vi "Get ID Collum.vi"(8 "error in (no error)":errorcluster caption="错误输入（无错误）", 11 "ExcelSave 输入":refnum<class "ExcelSave.lvclass"> caption="DNL_LabVIEW Object in") -> (0 "error out":errorcluster caption="错误输出", 1 "ID Row":i32, 2 "ID Collum":i32, 3 "ExcelSave 输出":refnum<class "ExcelSave.lvclass"> caption="DNL_LabVIEW Object out")   [LabVIEW 2016, in "ExcelSave.lvclass"]
uses:
  ExcelSave.lvclass
  ExcelSave.lvclass/ExcelSave.ctl
  <vilib>/Utility/NIReport.llb/NI_report.lvclass
  <vilib>/addons/_office/NI_ReportGenerationToolkit.lvlib
  <vilib>/Utility/NIReport.llb/Excel/NI_Excel.lvclass
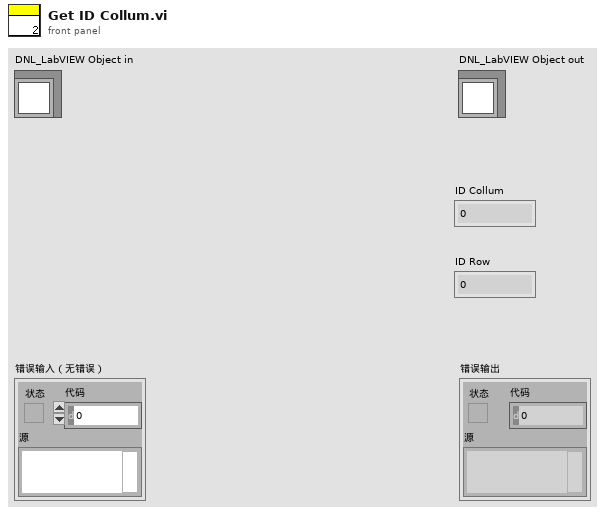
[diagram p1: front panel]
types:
  T1 = typedef "NI_ReportGenerationCore.lvlib/Report Data Members.ctl" = cluster{"font":T2, "from template?":bool}
  T2 = typedef "NI_ReportGenerationCore.lvlib/font.ctl" = cluster{"font name":string, "font size":dbl, "bold":u16, "italic":u16, "underline":u16, "strike through":u16, "font color":u32}
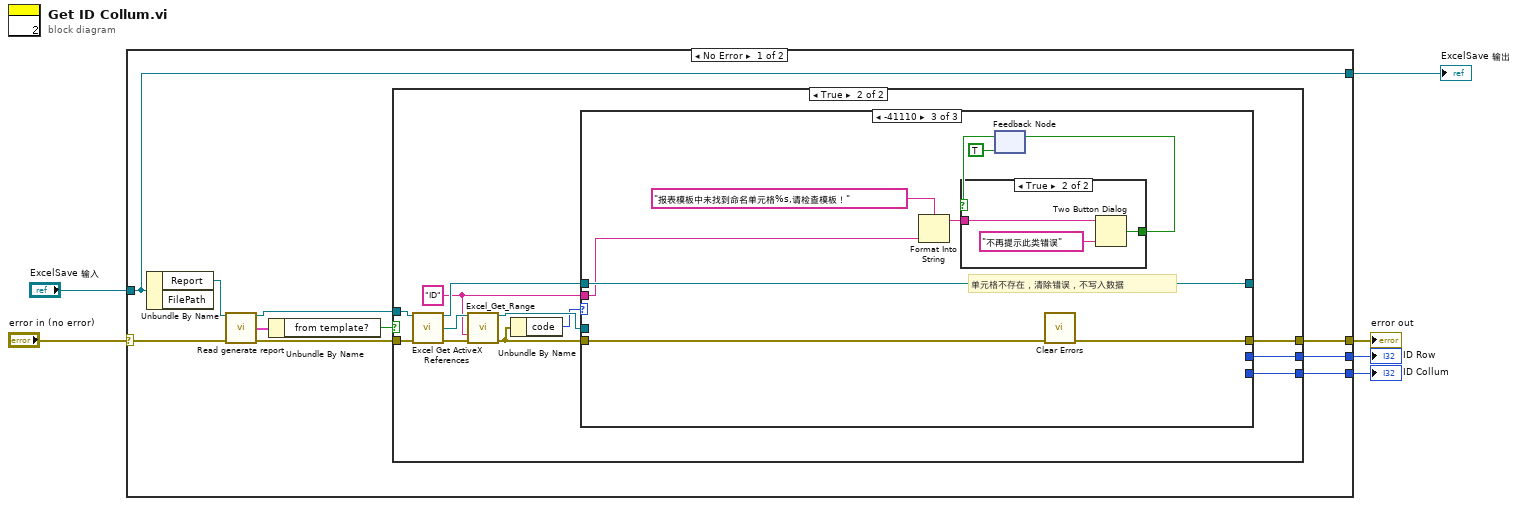
[diagram p0: block diagram]
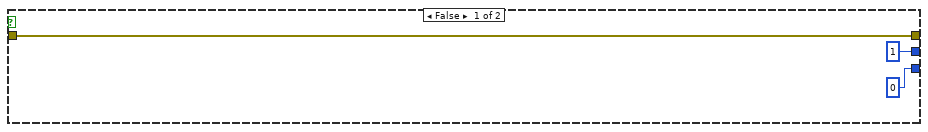
[diagram p2: hidden frame]
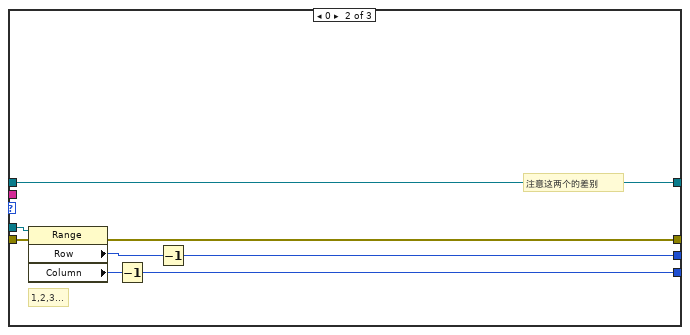
[diagram p4: hidden frame]
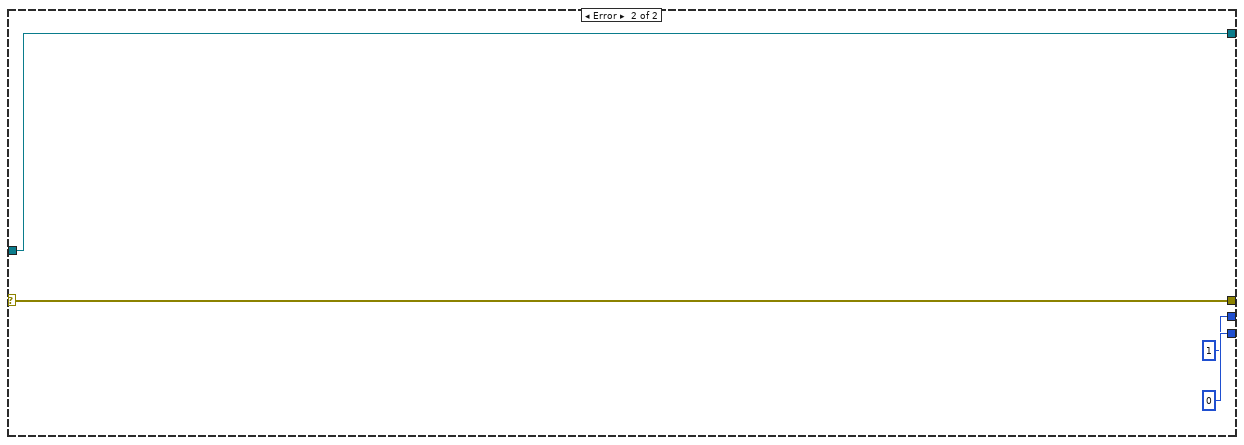
[diagram p6: hidden frame]
diagram:
  n1 = case shown="No Error" "error in (no error)" {
    selector: "error in (no error)" -> [w15 w57]
    tunnel: [w13 w58] -> w4
    tunnel: "ExcelSave 输入" -> [w13 w58]
    tunnel: [w9 w57] -> w3
    tunnel: [w8 0] -> w2
    tunnel: [w7 1] -> w1
    frame No Error {
      n2 = Unbundle By Name(w13) -> ("Report"=w16:refnum<class "NI_report.lvclass">)  [unwired: 1 out]
      n3 = call-dynamic "Read generate report.vi"("report in"=w16, "error in (no error)"=w15) -> ("report out"=w10:refnum<class "NI_report.lvclass">, "generate report"=w14:T1, "error out"=w12:errorcluster)  [unwired: 11 in]
      n4 = Unbundle By Name(w14) -> ("from template?"=w11:bool)
      n5 = case shown="True" w11 {
        tunnel: w12 -> [w19 w29]
        tunnel: w10 -> [_ w30]
        tunnel: [w19 w26] -> w9
        tunnel: [0 w22] -> w8
        tunnel: [1 w21] -> w7
        frame False {
        }
        frame True {
          w20 = "ID"
          n6 = call <vilib>:"Excel Get ActiveX References.vi"("report in"=w30, "error in (no error)"=w29) -> ("report out"=w27:refnum<class "NI_report.lvclass">, "Excel._Worksheet"=w31:refnum<k7>, "error out"=w28:errorcluster)  [unwired: 7 in, 4 out]
          n7 = call <vilib>:"Excel_Get_Range.vi"("Excel._Worksheet"=w31, "name"=w20, "error in (no error)"=w28) -> ("Range"=w24:refnum<k7>, "error out"=w25:errorcluster)  [unwired: 2 in, 9 out]
          n8 = Unbundle By Name(w25) -> ("code"=w23:i32)
          n9 = case shown="-41110" w23 {
            tunnel: w24 -> [_ w41 _]
            tunnel: w25 -> [w32 w40 w49]
            tunnel: w27 -> [w33 w37 w50]
            tunnel: [w33 w37 w50] -> _
            tunnel: [w32 w36 w48] -> w26
            tunnel: [_ w35 _] -> w22
            tunnel: [_ w34 _] -> w21
            tunnel: w20 -> [_ _ w42]
            frame 1, Default {
            }
            frame 0 {
              # "注意这两个的差别"
              # "1,2,3..."
              n10 = property class="Range"(reference=w41, error in=w40) -> (error out=w36:errorcluster, "Row"=w38:i32, "Column"=w39:i32)  [unwired: 1 out]
              n11 = Decrement(x=w39) -> (x-1=w35:i32)
              n12 = Decrement(x=w38) -> (x-1=w34:i32)
            }
            frame -41110 {
              # "单元格不存在，清除错误，不写入数据"
              n13 = Format Into String(format string="报表模板中未找到命名单元格%s,请检查模板！" ("格式字符串"), w42) -> (resulting string=w47:string)  [unwired: 2 in, 1 out]
              n14 = feedback #1(TRUE) -> (w43:bool)
              n15 = case shown="True" w43 {
                selector: w43 -> [w51 _]
                tunnel: w47 -> [_ w53]
                tunnel: [w51 w52] -> w44
                frame False {
                }
                frame True {
                  n16 = Two Button Dialog(message=w53, 1:"不再提示此类错误" ("F按钮名称（“取消”）")) -> (T button?=w52:bool)  [unwired: 1 in]
                }
              }
              n17 = feedback-in #1(w44) -> ()
              n18 = call <vilib>:"Clear Errors.vi"("error in (no error)"=w49) -> ("error out"=w48:errorcluster)  [unwired: 5 in, 1 out]
            }
          }
        }
      }
    }
    frame Error {
    }
  }
  "error out" <- w3
  "ExcelSave 输出" <- w4
  "ID Collum" <- w2
  "ID Row" <- w1
